vi "test_json_status.vi"() -> ()   [LabVIEW 2019]
panel:
  out "JSON string":string="{\"time\":\"2025-03-10T15:50:27.273Z\",\"hostComms\":false,\"topBoxComms\":false,\"AZPos\":0,\"AZPosReq\":0,\"AZPosError\":0,\"AZEncStatus\":0,\"AZLastRot\":\"\",\"mode\":\"\",\"modeReq\":\"\",\"subMode\":0,\"cmd\":0,\"buttons\":{\"EMStop\":false,\"forward\":false,\"reverse\":false,\"open\":false,\"close\":false,\"up\":false,\"down\":false,\"forceStop\":false},\"envSensor\":false,\"homed\":false,\"homing\":false,\"homeSensor\":false,\"config\":{\"cloudEn\":false,\"AZEncNeg\":false,\"AZEncRef\":0,\"AZEncStep\":0,\"homePos\":0,\"AZTimeout\":0,\"AZEncNoError\":0,\"posHSThreshold\":0,\"posTol\":0,\"cloudTimeout\":0,\"revDly\":0,\"AZEncCenter\":0,\"AZEncCenterThreshold\":0,\"AZEncCenterTol\":0,\"watchdogTim\":0,\"autoShutEn\":false,\"antWifi\":false},\"errors\":{\"EMStop\":false,\"AZEnc\":false,\"AZTimeout\":false,\"cloud\":false,\"M1\":false,\"M2\":false,\"M4\":false,\"watchdogTime\":false,\"shutdown\":false}}"
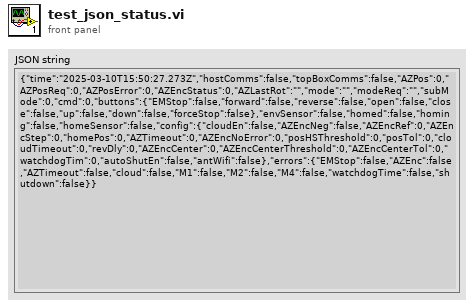
[diagram p1: front panel]
types:
  T1 = cluster{"time":string, "hostComms":bool, "topBoxComms":bool, "AZPos":dbl, "AZPosReq":dbl, "AZPosError":dbl, "AZEncStatus":u16, "AZLastRot":string, "mode":string, "modeReq":string, "subMode":u8, "cmd":i8, "buttons":cluster{"EMStop":bool, "forward":bool, "reverse":bool, "open":bool, "close":bool, "up":bool, "down":bool, "forceStop":bool}, "envSensor":bool, "homed":bool, "homing":bool, "homeSensor":bool, "config":cluster{"cloudEn":bool, "AZEncNeg":bool, "AZEncRef":u64, "AZEncStep":u64, "homePos":dbl, "AZTimeout":u32, "AZEncNoError":u16, "posHSThreshold":dbl, "posTol":dbl, "cloudTimeout":u32, "revDly":u32, "AZEncCenter":u64, "AZEncCenterThreshold":u64, "AZEncCenterTol":u64, "watchdogTim":i32, "autoShutEn":bool, "antWifi":bool}, "errors":cluster{"EMStop":bool, "AZEnc":bool, "AZTimeout":bool, "cloud":bool, "M1":bool, "M2":bool, "M4":bool, "watchdogTime":bool, "shutdown":bool}}
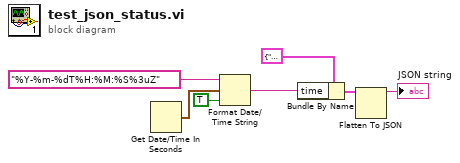
[diagram p0: block diagram]
diagram:
  n1 = Get Date/Time In Seconds() -> (seconds since 1Jan1904=w3:timestamp)
  n2 = Format Date/Time String(time format string (%c)="%Y-%m-%dT%H:%M:%S%3uZ", seconds (now)=w3, UTC format=TRUE) -> (date/time string=w2:string)
  n3 = Bundle By Name(cluster=T1 {"time"="", "hostComms"=FALSE, "topBoxComms"=FALSE, "AZPos"=0.0, "AZPosReq"=0.0, "AZPosError"=0.0, "AZEncStatus"=0, "AZLastRot"="", "mode"="", "modeReq"="", "subMode"=0, "cmd"=0, "buttons"={"EMStop"=FALSE, "forward"=FALSE, "reverse"=FALSE, "open"=FALSE, "close"=FALSE, "up"=FALSE, "down"=FALSE, "forceStop"=FALSE}, "envSensor"=FALSE, "homed"=FALSE, "homing"=FALSE, "homeSensor"=FALSE, "config"={"cloudEn"=FALSE, "AZEncNeg"=FALSE, "AZEncRef"=0, "AZEncStep"=0, "homePos"=0.0, "AZTimeout"=0, "AZEncNoError"=0, "posHSThreshold"=0.0, "posTol"=0.0, "cloudTimeout"=0, "revDly"=0, "AZEncCenter"=0, "AZEncCenterThreshold"=0, "AZEncCenterTol"=0, "watchdogTim"=0, "autoShutEn"=FALSE, "antWifi"=FALSE}, "errors"={"EMStop"=FALSE, "AZEnc"=FALSE, "AZTimeout"=FALSE, "cloud"=FALSE, "M1"=FALSE, "M2"=FALSE, "M4"=FALSE, "watchdogTime"=FALSE, "shutdown"=FALSE}} ("output cluster"), "time"=w2) -> (w6:T1)
  n4 = Flatten To JSON(anything=w6) -> (JSON string=→"JSON string":string)  [unwired: 2 in, 1 out]
